vi "SetZForInte_modify_Bmode_temperature_PRF&Volt.vi"(6 "meas_setting":T3={"measSetId"=6949, "measSetComments"="Orchid", "probeId"=141.0, "beamstyleIndex"=0, "txFrequencyHz"=3636400.0, "focusRangeCm"=8.0, "maxTxVoltageVolt"=100.0, "ceilTxVoltageVolt"=80.0, "profTxVoltageVolt"=62.0, "totalVoltagePt"=20, "numMeasVoltage"=12, "numTxElements"=118, "txpgWaveformStyle"=2, "numTxCycles"=4.0, "elevAperIndex"=0, "zStartDistCm"=1.5, "zMeasNum"=80, "IsTxAperModulationEn"=0, "DTxFreqIndex"=0, "VTxIndex"=0, "IsCPAEn"=0, "SysPulserSelA"=0, "TxPulseRleA"=""} {"zStartDistCm" format="%.2f"; "numTxCycles" format="%.1f"; "profTxVoltageVolt" format="%#_1g"; "ceilTxVoltageVolt" format="%.2f"; "maxTxVoltageVolt" format="%.2f"; "focusRangeCm" format="%.1f"; "txFrequencyHz" format="%.2f"}, 7 "timeout (ms)":dbl=40000.0 format="%.2f", 8 "error in (no error)":errorcluster, 9 "CW":bool, 10 "meas_temparature_Input":T2 {"scanRange" format="%.2f"; "numTxCycles" format="%#.2f"; "temperatureC" format="%.2f"; "pulseVoltage" format="%.2f"; "roomTempC" format="%.2f"}, 11 "TCP from Orchid in":refnum<k5>) -> (0 "error out":errorcluster, 1 "veri_P/F":bool, 2 "meas_temparature_Output":T1 {"scanRange" format="%.2f"; "temperatureC" format="%.2f"; "pulseVoltage" format="%.2f"; "roomTempC" format="%.2f"}, 3 "Actual PRF":dbl)   [LabVIEW 2016]
doc: "This VI sets the Z system transmit parameters for an intensity measurement, reads them back, and checks for errors. It first gets the initial center element delay (TxpgDelayAperA) and the system frequencies using tcpSysTxFreqFromZ.vi. It then sets the elevation aperture (using SetZElevAper.vi), channel modulation, wavestyle, frequency, focus, number of transmit elements, number of cycles, voltage, and voltage channel, in that order. It reads back the settings (using tcpReadIntenSettingsZ.vi) and checks for errors. The final trigger delay and change in delay, in microseconds, are calculated from the initial and final values of TxpgDelayAperA using:\ndelay(us) = (TxpgDelayAperA + 178.0) / 160"
uses:
  type def/measSetting.ctl
  GrobaLimitVoltage.vi
  TemperatureMeasure/Thermal_type.vi
panel:
  out "Receive array":string[](array[string])=["\r\n220 OK\r\nContainers within Hardware Control Layer\r\n\tHardwareModel\r\n\tHardwareControl\r\n\tHardwareAlgorithm\r\n\tSeq\r\n\tBeamforming\r\n\tDigitalReceiver\r\n\tEchoProcessor\r\n\tFlowProcessor\r\n\tHardwareScanConverter\r\n\tSip\r\n\tVideoInterface\r\n\tRtc\r\n\tCine\r\nScalar Parameters of Hardware Control Layer\r\nArray Parameters of Hardware Control Layer\r\ndebug\tDebug Functions\r\nquit\tExit DIOS\r\nback\tPrevious menu\r\nmain\tTop menu\r\nhelp\tAvailable commands\r\n\r\n", "\r\n220 OK\r\nContainers within Beamforming\r\n\tCommon\r\n\tBImage\r\n\tCbImage\r\n\tDImage\r\nScalar Parameters of Beamforming\r\nArray Parameters of Beamforming\r\ndebug\tDebug Functions\r\nquit\tExit DIOS\r\nback\tPrevious menu\r\nmain\tTop menu\r\nhelp\tAvailable commands\r\n\r\n", "\r\n220 OK\r\nContainers within Common\r\nScalar Parameters of Common\r\n\tBfPropagationVelCmPerSec\t154000\r\n\tDisUnit\t0.00385\r\n\tHwRcInterruptMask\t63\r\n\tHwRcTVP\t3\r\n\tHwRxAac0\t175\r\n\tHwRxAac1\t0\r\n\tHwRxbfBlankingWord\t0\r\n\tHwRxbfCmd1Word\t4232\r\n\tHwRxbfCmd2Word\t2\r\n\tHwRxbf0Cmd2Word\t3\r\n\tHwRxbfStartDelayWord\t10\r\n\tHwTiAttenuatorSelect\t0\r\n\tHwTiBitEn\t25088\r\n\tHwTiDacCtrl0\t255\r\n\tHwTiDacCtrl1\t2303\r\n\tHwTiDacCtrl2\t3327\r\n\tHwTiDacCtrl3\t511\r\n\tHwTiDacCtrl4\t2559\r\n\tHwTiDacCtrl5\t3583\r\n\tHwTiDacCtrl6\t767\r\n\tHwTiDacCtrl7\t2815\r\n\tHwTiDacCtrl8\t3839\r\n\tHwTiDacCtrl9\t2047\r\n\tHwTiDacCtrl10\t4095\r\n\tHwTiDigitalDriveCtrl\t0\r\n\tHwTiDigitalInterruptPolarity\t0\r\n\tHwTiDigitalReadCtrl\t0\r\n\tHwTiEchoBoosterCtrl\t0\r\n\tHwTiGlobalCtrl\t1\r\n\tHwTiHighVoltEn\t0\r\n\tHwTiInterruptClear\t65535\r\n\tHwTiInterruptMask\t32767\r\n\tHwTiMiscBitCtrl\t12\r\n\tHwTiProbeSelect\t2\r\n\tHwTiTXCLTransfer\t0\r\n\tHwTiVoltMultiplexer\t0\r\n\tHwTrGlobalCtrlAll\t1\r\n\tHwTrGlobalCtrl0All\t0\r\n\tHwTrDiagnosticCtrlAll\t0\r\n\tHwTrInterruptMaskAll\t1\r\n\tHwTrInterruptClearAll\t1\r\n\tHwTrRealTimeCtrlAll\t40\r\n\tHwTrTgcAacSignalCtrlAll\t0\r\n\tRxDelayRefx\t1\r\n\tRxDelayRefy\t-1\r\n\tTrPartNumber\t5928150\r\n\tBfPropagationVelFactor\t1\r\n\tDigitizingRateHz\t4e+007\r\n\tHwRxBfVectorLengthWord\t0\r\n\tIsRxVectorLengthEn\t1\r\n\tNumChannels\t192\r\n\tProbeBandwidthHz\t3.6e+006\r\n\tProbeId\t171\r\n\tProbeNumElem\t192\r\n\tProbeNumRows\t1\r\n\tProbePitchCm\t0.02\r\n\tProbeRadiusElectricalCm\t0\r\n\tProbeType\t0\r\n\tPropagationVelCmPerSec\t154000\r\n\tRxApod2dEn\t0\r\n\tRxbfAdcDelayClocks\t10\r\n\tRxbfGainShift\t0\r\n\tRxDelayYOffsetSysClk4\t0\r\n\tTxPulserMaxVolt\t50\r\nArray Parameters of Common\r\n\tHwRxbf0AdGainA\tsize=64\r\n\tHwRxbf1AdGainA\tsize=64\r\n\tHwRxbf2AdGainA\tsize=64\r\n\tHwRxbf3AdGainA\tsize=64\r\n\tHwRxbf4AdGainA\tsize=64\r\n\tHwRxbf5AdGainA\tsize=64\r\n\tHwRxbf6AdGainA\tsize=64\r\n\tHwRxbf7AdGainA\tsize=64\r\n\tHwRxbf8AdGainA\tsize=64\r\n\tHwRxbf9AdGainA\tsize=64\r\n\tHwRxbf10AdGainA\tsize=64\r\n\tHwRxbf11AdGainA\tsize=64\r\n\tHwRxAdOffsetCalA\tsize=192\r\n\tHwRxApodFilterRamA\tsize=512\r\n\tHwRxbf0DelayCalA\tsize=64\r\n\tHwRxbf1DelayCalA\tsize=64\r\n\tHwRxbf2DelayCalA\tsize=64\r\n\tHwRxbf3DelayCalA\tsize=64\r\n\tHwRxbf4DelayCalA\tsize=64\r\n\tHwRxbf5DelayCalA\tsize=64\r\n\tHwRxbf6DelayCalA\tsize=64\r\n\tHwRxbf7DelayCalA\tsize=64\r\n\tHwRxbf8DelayCalA\tsize=64\r\n\tHwRxbf9DelayCalA\tsize=64\r\n\tHwRxbf10DelayCalA\tsize=64\r\n\tHwRxbf11DelayCalA\tsize=64\r\n\tHwRxbf0DxA\tsize=64\r\n\tHwRxbf1DxA\tsize=64\r\n\tHwRxbf2DxA\tsize=64\r\n\tHwRxbf3DxA\tsize=64\r\n\tHwRxbf4DxA\tsize=64\r\n\tHwRxbf5DxA\tsize=64\r\n\tHwRxbf6DxA\tsize=64\r\n\tHwRxbf7DxA\tsize=64\r\n\tHwRxbf8DxA\tsize=64\r\n\tHwRxbf9DxA\tsize=64\r\n\tHwRxbf10DxA\tsize=64\r\n\tHwRxbf11DxA\tsize=64\r\n\tHwRxbf0DyA\tsize=64\r\n\tHwRxbf1DyA\tsize=64\r\n\tHwRxbf2DyA\tsize=64\r\n\tHwRxbf3DyA\tsize=64\r\n\tHwRxbf4DyA\tsize=64\r\n\tHwRxbf5DyA\tsize=64\r\n\tHwRxbf6DyA\tsize=64\r\n\tHwRxbf7DyA\tsize=64\r\n\tHwRxbf8DyA\tsize=64\r\n\tHwRxbf9DyA\tsize=64\r\n\tHwRxbf10DyA\tsize=64\r\n\tHwRxbf11DyA\tsize=64\r\n\tHwRxbf0DzA\tsize=128\r\n\tHwRxbf1DzA\tsize=128\r\n\tHwRxbf2DzA\tsize=128\r\n\tHwRxbf3DzA\tsize=128\r\n\tHwRxbf4DzA\tsize=128\r\n\tHwRxbf5DzA\tsize=128\r\n\tHwRxbf6DzA\tsize=128\r\n\tHwRxbf7DzA\tsize=128\r\n\tHwRxbf8DzA\tsize=128\r\n\tHwRxbf9DzA\tsize=128\r\n\tHwRxbf10DzA\tsize=128\r\n\tHwRxbf11DzA\tsize=128\r\n\tHwRxbf0PosInApodWinA\tsize=64\r\n\tHwRxbf1PosInApodWinA\tsize=64\r\n\tHwRxbf2PosInApodWinA\tsize=64\r\n\tHwRxbf3PosInApodWinA\tsize=64\r\n\tHwRxbf4PosInApodWinA\tsize=64\r\n\tHwRxbf5PosInApodWinA\tsize=64\r\n\tHwRxbf6PosInApodWinA\tsize=64\r\n\tHwRxbf7PosInApodWinA\tsize=64\r\n\tHwRxbf8PosInApodWinA\tsize=64\r\n\tHwRxbf9PosInApodWinA\tsize=64\r\n\tHwRxbf10PosInApodWinA\tsize=64\r\n\tHwRxbf11PosInApodWinA\tsize=64\r\n\tHwRxMuxSelectLutA\tsize=512\r\n\tHwRxRamOffsetA\tsize=12\r\n\tHwTxDacA\tsize=2\r\n\tHwTxpgDelayAperA\tsize=393216\r\n\tNumBitsPerCycleA\tsize=49\r\n\tNumCyclesPerPassA\tsize=49\r\n\tNumWordsPerPassA\tsize=49\r\n\tRxAdGainA\tsize=256\r\n\tRxDelayCalA\tsize=768\r\n\tRxDxA\tsize=256\r\n\tRxDyA\tsize=256\r\n\tRxDzA\tsize=256\r\n\tRxMuxSelectLutPtrA\tsize=512\r\n\tRxPosInApodWinA\tsize=768\r\n\tTxDelayCalA\tsize=192\r\n\tTxpgWaveformHoutA\tsize=15680\r\n\tTxpgWaveformLoutA\tsize=15680\r\n\tYIndexTableA\tsize=256\r\n\tZIndexTableA\tsize=256\r\n\tInsertedProbeIdA\tsize=6\r\n\tPulseVoltageA\tsize=2\r\n\tRxApodFactorA\tsize=4\r\n\tRxApodSelA\tsize=4\r\n\tSysTxFreqHzA\tsize=49\r\ndebug\tDebug Functions\r\nquit\tExit DIOS\r\nback\tPrevious menu\r\nmain\tTop menu\r\nhelp\tAvailable commands\r\n\r\n", "220 OK\r\n", "250 20\r\n"]
  out "error out 2":errorcluster
  out "Pass_count":i16
  out "All_param_veri":bool[](array[boolean])
  in  "volt channel":i8
  # "Program constants"
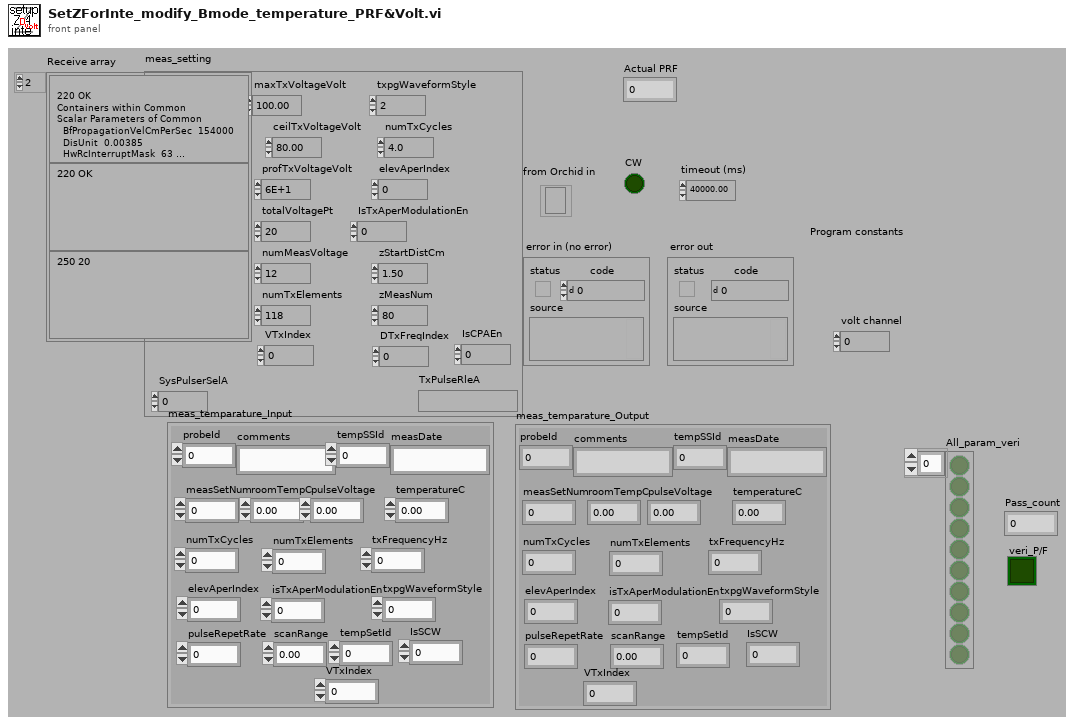
[diagram p1: front panel]
types:
  T1 = cluster{"probeId":sgl, "comments":string, "tempSSId":i16, "measDate":string, "measSetNum":i16, "roomTempC":sgl, "pulseVoltage":dbl, "temperatureC":ext, "numTxCycles":dbl, "numTxElements":i16, "txFrequencyHz":i32, "elevAperIndex":i16, "isTxAperModulationEn":i16, "txpgWaveformStyle":i16, "pulseRepetRate":i32, "scanRange":dbl, "tempSetId":i16, "IsSCW":i16, "VTxIndex":i16}
  T2 = cluster{"probeId":sgl, "comments":string, "tempSSId":i16, "measDate":string, "measSetNum":i16, "roomTempC":sgl, "pulseVoltage":dbl, "temperatureC":ext, "numTxCycles":dbl, "numTxElements":i16, "txFrequencyHz":i32, "elevAperIndex":i16, "isTxAperModulationEn":i16, "txpgWaveformStyle":i16, "pulseRepetRate":dbl, "scanRange":dbl, "tempSetId":i16, "IsSCW":i16, "VTxIndex":i16}
  T3 = typedef "measSetting.ctl" = cluster{"measSetId":i32, "measSetComments":string, "probeId":sgl, "beamstyleIndex":i16, "txFrequencyHz":sgl, "focusRangeCm":sgl, "maxTxVoltageVolt":sgl, "ceilTxVoltageVolt":sgl, "profTxVoltageVolt":dbl, "totalVoltagePt":i8, "numMeasVoltage":i8, "numTxElements":i16, "txpgWaveformStyle":i8, "numTxCycles":sgl, "elevAperIndex":i8, "zStartDistCm":sgl, "zMeasNum":i8, "IsTxAperModulationEn":i8, "DTxFreqIndex":i16, "VTxIndex":i8, "IsCPAEn":i16, "SysPulserSelA":i16, "TxPulseRleA":string}
  T4 = cluster{"pulseVoltage":dbl, "numTxCycles":dbl, "numTxElements":i16, "txFrequencyIndex":i32, "isTxAperModulationEn":i16, "txpgWaveformStyle":i16, "pulseRepetRate":dbl, "FocalRangeCm":dbl, "RoiLateralSpan":dbl, "RoiLateralMin":dbl}
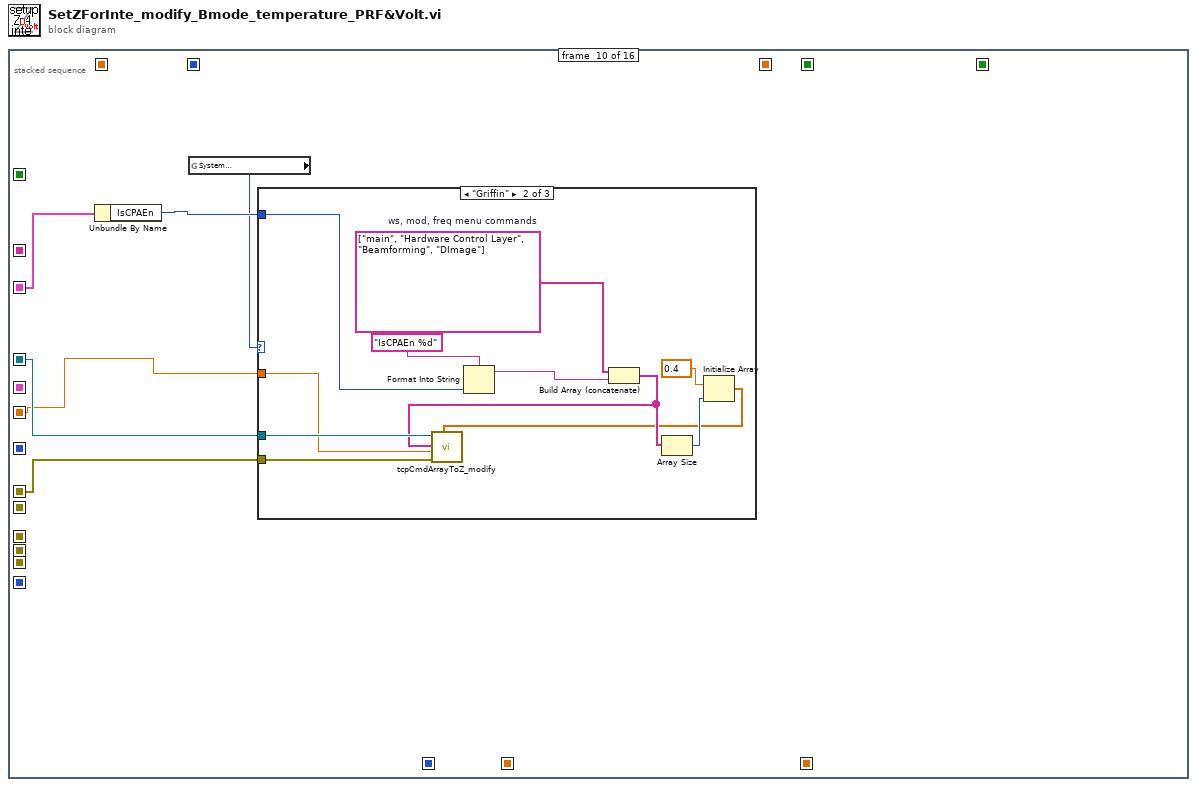
[diagram p0: block diagram]
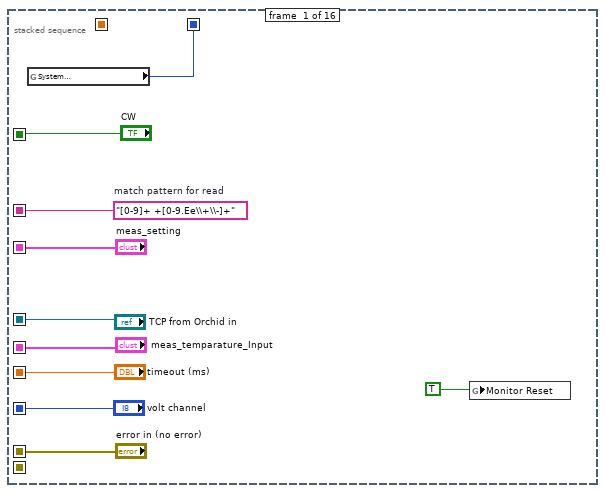
[diagram p2: hidden frame]
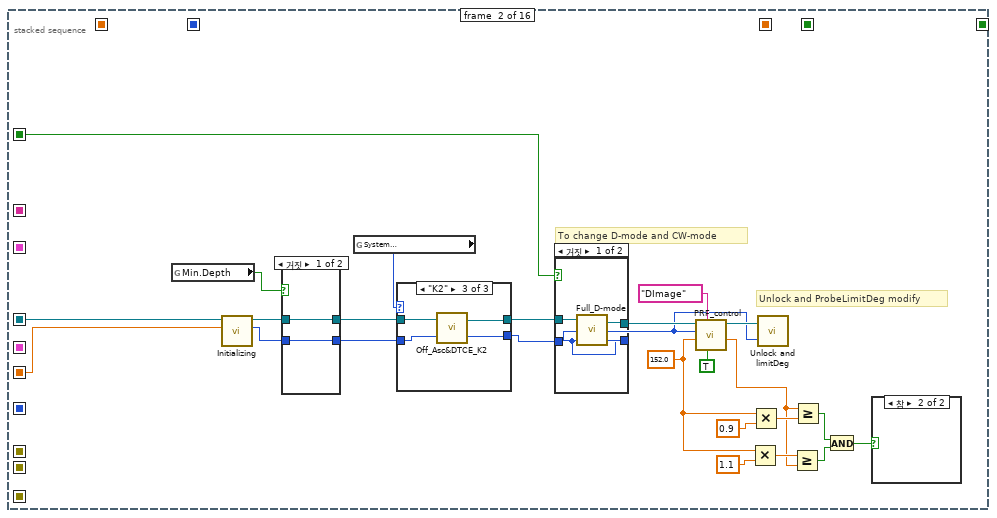
[diagram p3: hidden frame]
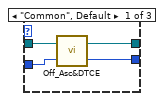
[diagram p4: hidden frame]
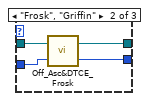
[diagram p5: hidden frame]
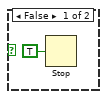
[diagram p6: hidden frame]
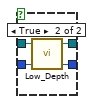
[diagram p7: hidden frame]
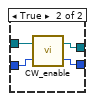
[diagram p8: hidden frame]
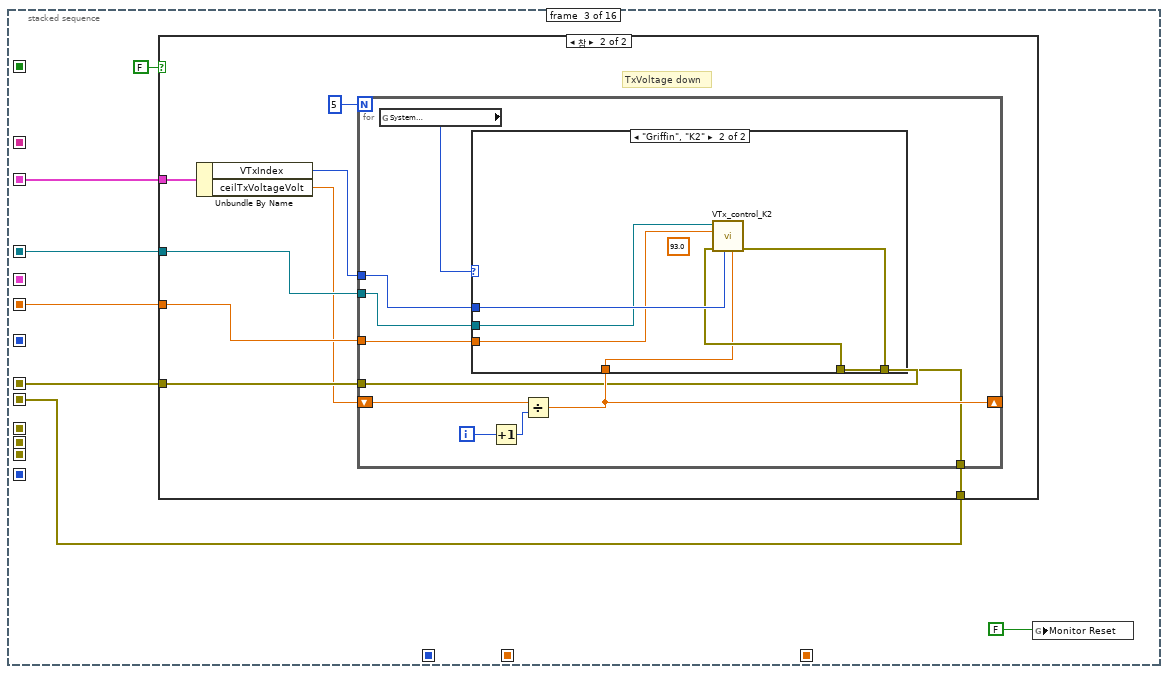
[diagram p9: hidden frame]
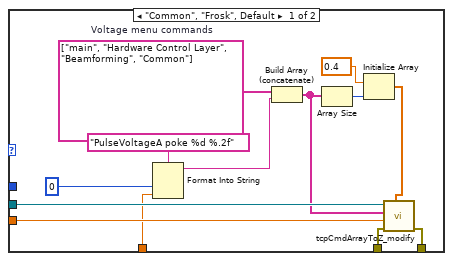
[diagram p11: hidden frame]
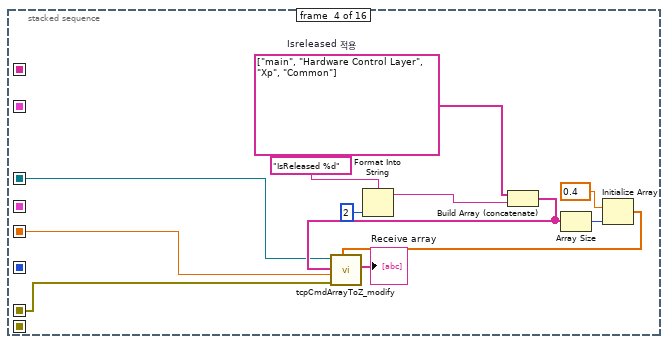
[diagram p12: hidden frame]
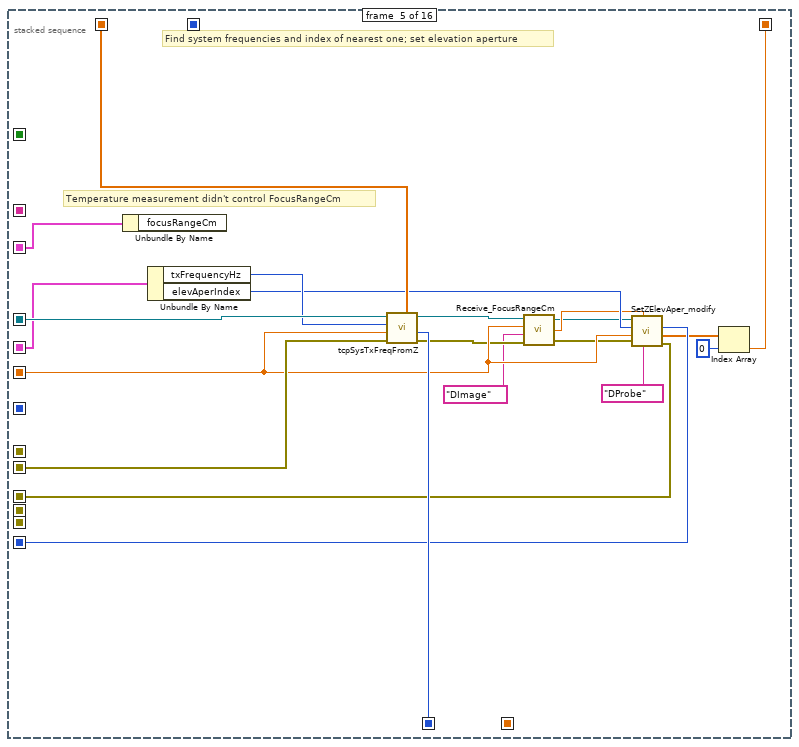
[diagram p13: hidden frame]
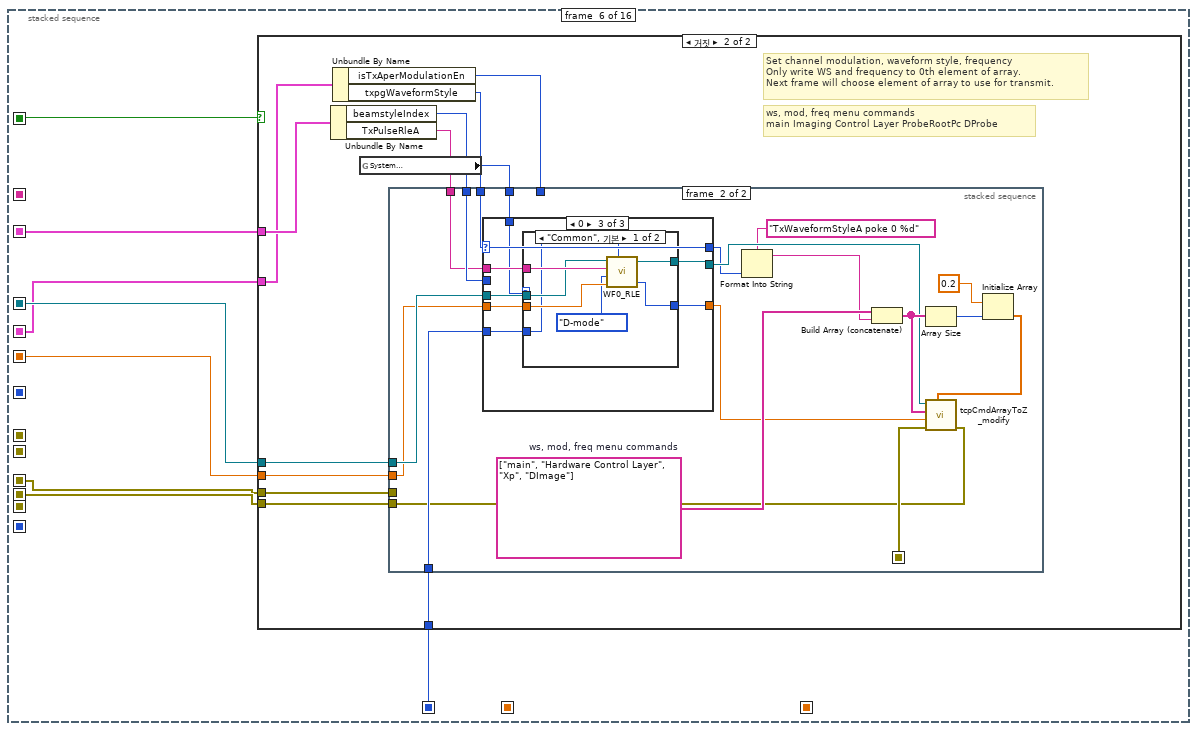
[diagram p14: hidden frame]
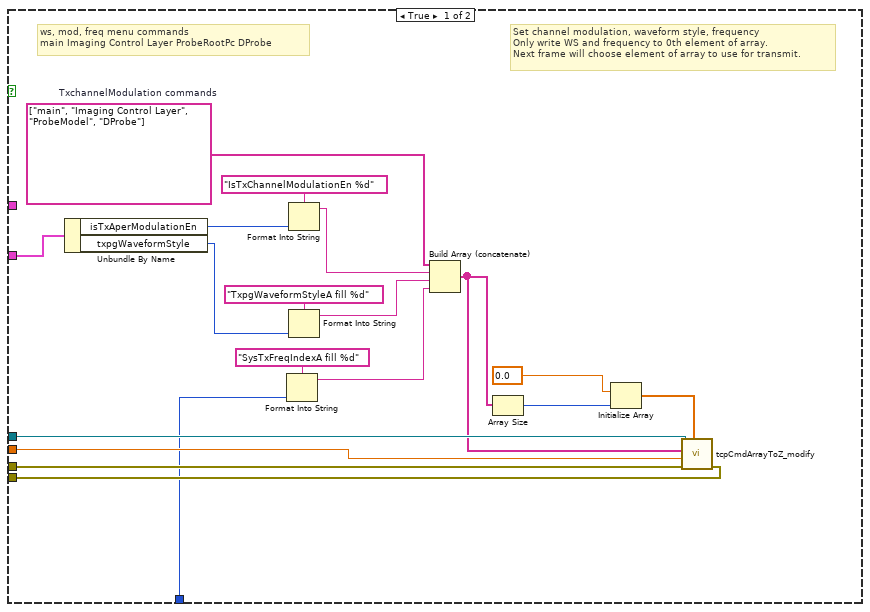
[diagram p15: hidden frame]
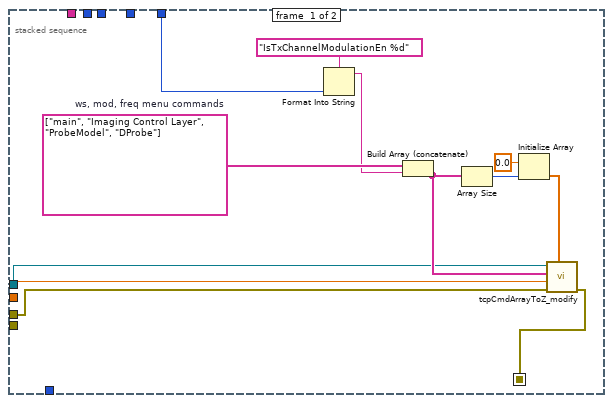
[diagram p16: hidden frame]
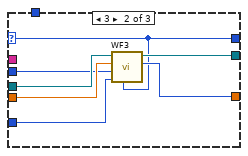
[diagram p18: hidden frame]
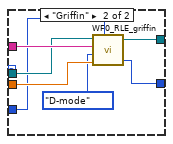
[diagram p19: hidden frame]
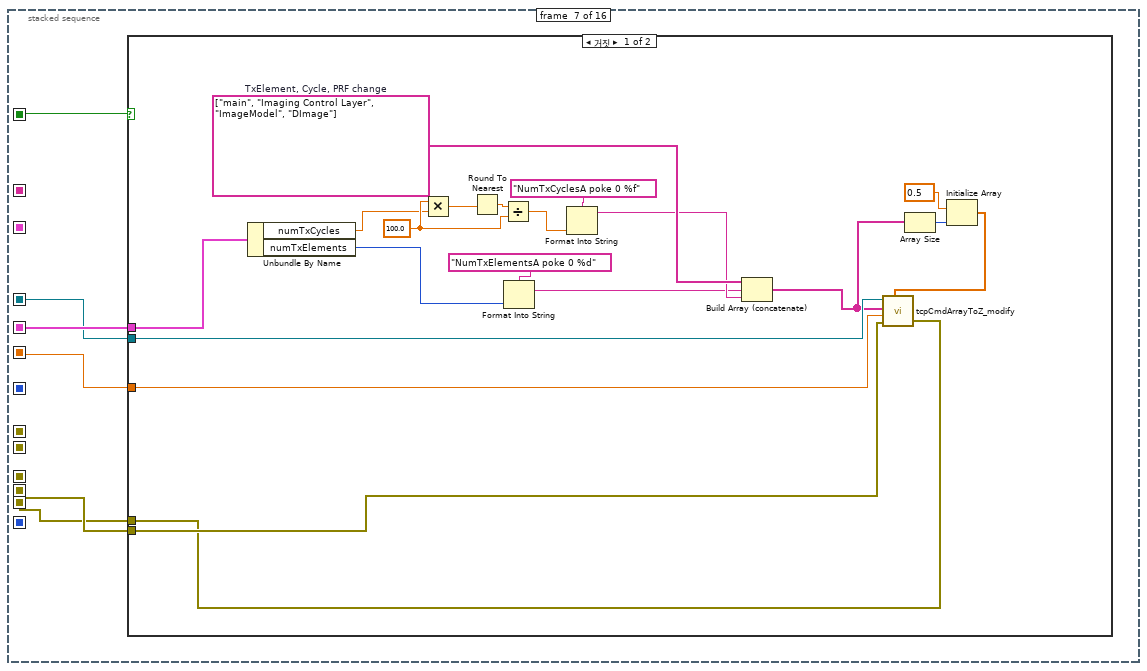
[diagram p20: hidden frame]
diagram:
  n1 = stacked-sequence {
    seq-local: ["meas_temparature_Input" _ _ _ _ _ _ _ _ _ _ _ _ _ _ _] -> [_ _ _ _ w138 w142 w247 w293 _ _ _ w394 w465 _ _ _]
    seq-local: ["TCP from Orchid in" _ _ _ _ _ _ _ _ _ _ _ _ _ _ _] -> [_ w35 w68 w109 w139 w147 w245 w281 w296 w311 w339 w396 w458 w509 w518 w525]
    seq-local: ["timeout (ms)" _ _ _ _ _ _ _ _ _ _ _ _ _ _ _] -> [_ w34 w67 w107 w124 w146 w244 w279 w295 w310 w337 w395 w457 w508 w517 w524]
    seq-local: [_ _ _ _ w133 _ _ _ _ _ _ _ _ _ _ _] -> [_ _ _ _ _ w144 _ _ _ _ _ _ _ _ _ _]
    seq-local: [_ _ _ _ w137 _ _ _ _ _ _ _ _ _ _ _] -> [_ _ _ _ _ _ _ _ _ _ _ _ _ _ _ _]
    seq-local: ["volt channel" _ _ _ _ _ _ _ _ _ _ _ _ _ _ _] -> [_ _ _ _ _ _ _ _ _ _ _ _ _ _ _ _]
    seq-local: ["error in (no error)" _ _ _ _ _ _ _ _ _ _ _ _ _ _ _] -> [_ _ w64 w108 _ _ _ _ _ w309 w338 w414 _ _ _ _]
    seq-local: [w7 _ _ _ _ _ _ _ _ _ _ _ _ _ _ _] -> [_ _ _ _ _ _ _ _ _ _ _ _ _ _ _ _]
    seq-local: [_ _ w63 _ _ _ _ _ _ _ _ _ _ _ _ _] -> [_ _ _ _ w134 _ _ _ _ _ _ _ _ _ _ _]
    seq-local: [_ _ _ _ _ w145 _ _ _ _ _ _ _ _ _ _] -> [_ _ _ _ _ _ w246 _ _ _ _ _ _ _ _ _]
    seq-local: [_ _ _ _ _ _ w243 _ _ _ _ _ _ _ _ _] -> [_ _ _ _ _ _ _ _ _ _ _ _ w456 w504 _ _]
    seq-local: ["meas_setting" _ _ _ _ _ _ _ _ _ _ _ _ _ _ _] -> [_ _ w66 _ w126 w140 _ _ _ w308 _ w393 w460 _ _ _]
    seq-local: ["CW" _ _ _ _ _ _ _ _ _ _ _ _ _ _ _] -> [_ w31 _ _ _ w143 w242 _ _ _ _ w397 w451 _ _ _]
    seq-local: [_ _ _ _ w135 _ _ _ _ _ _ _ _ _ _ _] -> [_ _ _ _ _ w141 _ _ w297 _ _ w412 _ _ _ _]
    seq-local: [_ _ _ _ _ _ _ _ _ _ _ w386 _ _ _ _] -> [_ _ _ _ _ _ _ _ _ _ _ _ _ w507 _ _]
    seq-local: [_ _ _ _ _ _ _ w280 _ _ _ _ _ _ _ _] -> [_ _ _ _ _ _ _ _ _ _ _ w413 _ _ _ _]
    seq-local: [_ _ _ _ _ _ _ _ _ _ _ _ w453 _ _ _] -> [_ _ _ _ _ _ _ _ _ _ _ _ _ w506 _ _]
    seq-local: [_ _ _ _ w130 _ _ _ _ _ _ _ _ _ _ _] -> [_ _ _ _ _ _ _ _ _ _ _ w385 _ _ _ _]
    seq-local: [_ _ _ _ w127 _ _ _ _ _ _ _ _ _ _ _] -> [_ _ _ _ _ _ _ _ _ _ _ w384 _ _ _ _]
    seq-local: [w1 _ _ _ _ _ _ _ _ _ _ _ _ _ _ _] -> [_ _ _ _ _ _ _ _ w294 _ _ w390 w452 _ _ _]
    seq-local: [_ _ _ _ _ _ _ _ _ _ w335 _ _ _ _ _] -> [_ _ _ _ _ _ _ _ _ _ _ w367 _ _ _ _]
    frame #0 {
      w7 = "[0-9]+ +[0-9.Ee\\+\\-]+"  # match pattern for read
      n2 = global read "Thermal_type.vi" "System \nSelection"() -> (w1:enum32{"Common", "Frosk", "Griffin", "K2"})
      n3 = global write "GrobaLimitVoltage.vi" "Monitor Reset"(TRUE) -> ()
    }
    frame #1 {
      w20 = 152.0 ("Input PRF")
      # "Unlock and ProbeLimitDeg modify"
      # "To change D-mode and CW-mode"
      n4 = global read "Thermal_type.vi" "Min.Depth"() -> (w30:bool)
      n5 = call "Initializing.vi"("Timeout (ms)"=w34, "connection ID in"=w35) -> ("Timeout (ms) 2"=w32:i32, "connection ID in 2"=w33:refnum<k5>)  [unwired: 8 in]
      n6 = case shown="거짓" w30 {
        tunnel: w33 -> [w50 w54]
        tunnel: w32 -> [w49 w53]
        tunnel: [w50 w52] -> w14
        tunnel: [w49 w51] -> w13
        frame False {
        }
        frame True {
          n7 = call "Low_Depth.vi"("Timeout (ms)"=w53, "connection ID in"=w54) -> ("Timeout (ms) 2"=w51:i32, "connection ID out"=w52:refnum<k5>)  [unwired: 2 in]
        }
      }
      n8 = global read "Thermal_type.vi" "System \nSelection"() -> (w15:enum32{"Common", "Frosk", "Griffin", "K2"})
      n9 = case shown="\"K2\"" w15 {
        tunnel: [w39 w43 w45] -> w12
        tunnel: [w38 w42 w44] -> w11
        tunnel: w14 -> [w37 w41 w47]
        tunnel: w13 -> [w36 w40 w46]
        frame "Common", Default {
          n10 = call "Off_Asc&DTCE.vi"("Timeout (ms)"=w36, "connection ID in"=w37) -> ("Timeout (ms) 2"=w38:i32, "connection ID out"=w39:refnum<k5>)
        }
        frame "Frosk", "Griffin" {
          n11 = call "Off_Asc&DTCE_Frosk.vi"("Timeout (ms)"=w40, "connection ID in"=w41) -> ("Timeout (ms) 2"=w42:i32, "connection ID out"=w43:refnum<k5>)
        }
        frame "K2" {
          n12 = call "Off_Asc&DTCE_K2.vi"("Timeout (ms)"=w46, "connection ID in"=w47) -> ("Timeout (ms) 2"=w44:i32, "connection ID out"=w45:refnum<k5>)
        }
      }
      n13 = case shown="거짓" w31 {
        tunnel: w12 -> [w57 w61]
        tunnel: w11 -> [w55 w60]
        tunnel: [w56 w59] -> w19
        tunnel: [w55 w58] -> w17
        frame False {
          n14 = call "Full_D-mode.vi"("Timeout (ms) 입력"=w55, "TCP 네트워크 연결 입력"=w57) -> ("TCP 네트워크 연결 출력"=w56:refnum<k5>)  [unwired: 1 in]
        }
        frame True {
          n15 = call "CW_enable.vi"("Timeout (ms)"=w60, "connection ID in"=w61) -> ("Timeout (ms) 2"=w58:i32, "connection ID out"=w59:refnum<k5>)
        }
      }
      n16 = call "PRF_control.vi"("PRF_Event Down"=TRUE, "mode selection"="DImage", "Input PRF"=w20, "timeout (ms)"=w17, "TCP from Orchid in"=w19) -> ("PRF"=w21:dbl, "connection ID out"=w18:refnum<k5>)  [unwired: 2 in, 1 out]
      n17 = Multiply(x=w20, y=1.1) -> (x*y=w26:dbl)
      n18 = Multiply(x=w20, y=0.9) -> (x*y=w22:dbl)
      n19 = call "Unlock and limitDeg.vi"("Timeout (ms)"=w17, "connection ID in"=w18) -> ()  [unwired: 2 out]
      n20 = Greater Or Equal?(x=w26, y=w21) -> (x >= y?=w25:bool)
      n21 = Greater Or Equal?(x=w21, y=w22) -> (x >= y?=w24:bool)
      n22 = And(x=w24, y=w25) -> (x .and. y?=w23:bool)
      n23 = case shown="참" w23 {
        frame False {
          n24 = Stop(stop? (T)=TRUE ("정지? (참)")) -> ()
        }
        frame True {
        }
      }
    }
    frame #2 {
      n25 = case shown="참" FALSE {
        tunnel: w68 -> [_ w77]
        tunnel: w67 -> [_ w76]
        tunnel: w66 -> [_ w75]
        tunnel: w64 -> [w69 w72]
        tunnel: [w69 w71] -> w63
        frame False {
        }
        frame True {
          # "TxVoltage down"
          n26 = Unbundle By Name(w75) -> ("VTxIndex"=w73:i8, "ceilTxVoltageVolt"=w70:sgl)
          n27 = for {
            N: 5 -> [_]
            tunnel: w77 -> [w87]
            tunnel: w76 -> [w86]
            shift-right: [w80] -> _
            shift-left: w70 -> [w82]
            tunnel: w73 -> [w85]
            tunnel: w72 -> [w79]
            tunnel: [w78] -> w71
            i -> [w81]
            n28 = global read "Thermal_type.vi" "System \nSelection"() -> (w84:enum32{"Common", "Frosk", "Griffin", "K2"})
            n29 = Increment(x=w81) -> (x+1=w83:i32)
            n30 = Divide(x=w82, y=w83) -> (x/y=w80:sgl)
            n31 = case shown="\"Griffin\", \"K2\"" w84 {
              tunnel: w87 -> [w100 w105]
              tunnel: w86 -> [w99 w104]
              tunnel: w85 -> [_ w106]
              tunnel: w80 -> [w90 w101]
              tunnel: w79 -> [w89 w103]
              tunnel: [w88 w102] -> w78
              frame "Common", "Frosk", Default {
                w97 = string[] ["main", "Hardware Control Layer", "Beamforming", "Common"]  # Voltage menu commands
                n32 = Format Into String(format string="PulseVoltageA poke %d %.2f" ("Format String"), i8 0 ("입력 1"), w90) -> (resulting string=w96:string)  [unwired: 2 in, 1 out]
                n33 = Build Array (concatenate)(w97, w96) -> (w92:string[])
                n34 = Array Size(array=w92) -> (size(s)=w95:i32)
                n35 = Initialize Array(0.4 ("element"), w95) -> (w93:dbl[])
                n36 = call "tcpCmdArrayToZ_modify.vi"("Delay (sec)"=w93, "error in (no error)"=w89, "Timeout (ms)"=w99, "Command array"=w92, "connection ID in"=w100) -> ("error out"=w88:errorcluster)  [unwired: 2 in, 4 out]
              }
              frame "Griffin", "K2" {
                (unwired) 93.0 ("VTx1_voltage")
                n37 = call "VTx_control_K2.vi"("VTx_Voltage"=w101, "VTxIndex_In"=w106, "error in (no error)"=w103, "Timeout (ms)"=w104, "connection ID in"=w105) -> ("error out"=w102:errorcluster)  [unwired: 5 in, 1 out]
              }
            }
          }
        }
      }
      n38 = global write "GrobaLimitVoltage.vi" "Monitor Reset"(FALSE) -> ()
    }
    frame #3 {
      w112 = string[] ["main", "Hardware Control Layer", "Xp", "Common"]  # Isreleased 적용
      n39 = Format Into String(format string="IsReleased %d" ("Format String"), i16 2 ("입력 1")) -> (resulting string=w117:string)  [unwired: 2 in, 1 out]
      n40 = Build Array (concatenate)(w112, w117) -> (w114:string[])
      n41 = Array Size(array=w114) -> (size(s)=w116:i32)
      n42 = Initialize Array(0.4 ("element"), w116) -> (w113:dbl[])
      n43 = call "tcpCmdArrayToZ_modify.vi"("Delay (sec)"=w113, "error in (no error)"=w108, "Timeout (ms)"=w107, "Command array"=w114, "connection ID in"=w109) -> ("Receive array"=→"Receive array":string[])  [unwired: 2 in, 4 out]
    }
    frame #4 {
      # "Temperature measurement didn't control FocusRangeCm"
      # "Find system frequencies and index of nearest one; set elevation aperture"
      n44 = Unbundle By Name(w126) -> ()  [unwired: 1 out]
      n45 = Unbundle By Name(w138) -> ("txFrequencyHz"=w136:i32, "elevAperIndex"=w132:i16)
      n46 = call "tcpSysTxFreqFromZ.vi"("error in (no error)"=w134, "timeout (ms)"=w124, "txFrequencyHz in"=w136, "connection ID in"=w139) -> ("error out"=w123:errorcluster, "TxFreqIndex"=w135:i8, "connection ID out"=w121:refnum<k5>, "SysTxFreqHzA"=w137:sgl[])  [unwired: 3 in, 1 out]
      n47 = call "Receive_FocusRangeCm.vi"("error in (no error)"=w123, "Image mode"="DImage", "Timeout (ms)"=w124, "connection ID in"=w121) -> ("error out"=w122:errorcluster, "FocusRangeCm"=w125:dbl, "connection ID out"=w120:refnum<k5>)
      n48 = call "SetZElevAper_modify.vi"("Mode"="DProbe", "focusRangeCm"=w125, "error in (no error)"=w122, "timeout (ms)"=w124, "elevAperIndex"=w132, "connection ID in"=w120) -> ("error out"=w133:errorcluster, "SwitchDepth"=w129:sgl[], "probeNumElevAper"=w130:i32)  [unwired: 2 in, 1 out]
      n49 = Index Array(array=w129, index=0 ("인덱스")) -> (element=w127:sgl)
    }
    frame #5 {
      n50 = case shown="거짓" w143 {
        tunnel: w147 -> [w166 w176]
        tunnel: w146 -> [w165 w175]
        tunnel: [w163 w169] -> w145
        tunnel: w144 -> [w162 w178]
        tunnel: w142 -> [w160 w173]
        tunnel: w141 -> [w149 w177]
        tunnel: w140 -> [_ w174]
        frame True {
          w155 = string[] ["main", "Imaging Control Layer", "ProbeModel", "DProbe"]  # TxchannelModulation commands
          # "ws, mod, freq menu commands\nmain Imaging Control Layer ProbeRootPc DProbe"
          # "Set channel modulation, waveform style, frequency\nOnly write WS and frequency to 0th element of array.\nNext frame will choose element of array to use for transmit."
          n51 = Unbundle By Name(w160) -> ("isTxAperModulationEn"=w161:i16, "txpgWaveformStyle"=w153:i16)
          n52 = Format Into String(format string="SysTxFreqIndexA fill %d" ("Format String"), w149) -> (resulting string=w148:string)  [unwired: 2 in, 1 out]
          n53 = Format Into String(format string="IsTxChannelModulationEn %d" ("Format String"), w161) -> (resulting string=w154:string)  [unwired: 2 in, 1 out]
          n54 = Format Into String(format string="TxpgWaveformStyleA fill %d" ("Format String"), w153) -> (resulting string=w152:string)  [unwired: 2 in, 1 out]
          n55 = Build Array (concatenate)(w155, w154, w152, w148) -> (w159:string[])
          n56 = Array Size(array=w159) -> (size(s)=w158:i32)
          n57 = Initialize Array(0.0 ("element"), w158) -> (w156:dbl[])
          n58 = call "tcpCmdArrayToZ_modify.vi"("Delay (sec)"=w156, "error in (no error)"=w162, "Timeout (ms)"=w165, "Command array"=w159, "connection ID in"=w166) -> ("error out"=w163:errorcluster)  [unwired: 2 in, 4 out]
        }
        frame False {
          # "ws, mod, freq menu commands\nmain Imaging Control Layer ProbeRootPc DProbe"
          # "Set channel modulation, waveform style, frequency\nOnly write WS and frequency to 0th element of array.\nNext frame will choose element of array to use for transmit."
          n59 = Unbundle By Name(w174) -> ("beamstyleIndex"=w170:i16, "TxPulseRleA"=w168:string)
          n60 = Unbundle By Name(w173) -> ("isTxAperModulationEn"=w172:i16, "txpgWaveformStyle"=w171:i16)
          n61 = global read "Thermal_type.vi" "System \nSelection"() -> (w167:enum32{"Common", "Frosk", "Griffin", "K2"})
          n62 = stacked-sequence {
            seq-local: [w179 _] -> [_ w195]
            tunnel: w178 -> [w180 _]
            tunnel: w177 -> [_ w199]
            tunnel: w176 -> [w183 w204]
            tunnel: w175 -> [w182 w201]
            tunnel: w172 -> [w181 _]
            tunnel: w171 -> [_ w193]
            tunnel: w170 -> [_ w200]
            tunnel: [_ w194] -> w169
            tunnel: w168 -> [_ w192]
            tunnel: w167 -> [_ w191]
            frame #0 {
              w189 = string[] ["main", "Imaging Control Layer", "ProbeModel", "DProbe"]  # ws, mod, freq menu commands
              n63 = Format Into String(format string="IsTxChannelModulationEn %d" ("Format String"), w181) -> (resulting string=w188:string)  [unwired: 2 in, 1 out]
              n64 = Build Array (concatenate)(w189, w188) -> (w185:string[])
              n65 = Array Size(array=w185) -> (size(s)=w186:i32)
              n66 = Initialize Array(sgl 0.0 ("Element Data"), w186) -> (w184:sgl[])
              n67 = call "tcpCmdArrayToZ_modify.vi"("Delay (sec)"=w184, "error in (no error)"=w180, "Timeout (ms)"=w182, "Command array"=w185, "connection ID in"=w183) -> ("error out"=w179:errorcluster)  [unwired: 2 in, 4 out]
            }
            frame #1 {
              w209 = string[] ["main", "Hardware Control Layer", "Xp", "DImage"]  # ws, mod, freq menu commands
              n68 = case shown="0" w193 {
                selector: w193 -> [w210 w213 w222]
                tunnel: w204 -> [w212 w219 w226]
                tunnel: [w212 w218 w223] -> w203
                tunnel: [w211 w217 w224] -> w202
                tunnel: w201 -> [w211 w216 w225]
                tunnel: w200 -> [_ w215 _]
                tunnel: w199 -> [_ w214 w221]
                tunnel: [w210 w213 w222] -> w197
                tunnel: w192 -> [_ _ w227]
                tunnel: w191 -> [_ _ w220]
                frame Default {
                }
                frame 3 {
                  n69 = call "WF3.vi"("TxWaveformStyle"=w213, "TxFreqIndex"=w214, "BeamStyleIndex"=w215, "Timeout (ms)"=w216, "connection ID in"=w219) -> ("Timeout (ms) out"=w217:i32, "connection ID out"=w218:refnum<k5>)  [unwired: 5 in]
                }
                frame 0 {
                  n70 = case shown="\"Common\", 기본" w220 {
                    tunnel: w227 -> [w234 w241]
                    tunnel: w226 -> [w233 w240]
                    tunnel: w225 -> [w232 w239]
                    tunnel: [w231 w238] -> w224
                    tunnel: [w230 w237] -> w223
                    tunnel: w221 -> [w228 w235]
                    frame "Common", Default {
                      n71 = call "WF0_RLE.vi"("connection ID in"=w233, "TxPulseRleA"=w234, "Mode control"=enum32{"D-mode", "B-mode"}."D-mode", "Timeout (ms)"=w232, "TxFrequencyIndex"=w228) -> ("connection ID out"=w230:refnum<k5>, "Timeout (ms) out"=w231:i32)  [unwired: 1 in]
                    }
                    frame "Griffin" {
                      n72 = call "WF0_RLE_griffin.vi"("connection ID in"=w240, "TxPulseRleA"=w241, "Mode control"=enum32{"D-mode", "B-mode"}."D-mode", "Timeout (ms)"=w239, "TxFrequencyIndex"=w235) -> ("connection ID out"=w237:refnum<k5>, "Timeout (ms) out"=w238:i32)  [unwired: 1 in]
                    }
                  }
                }
              }
              n73 = Format Into String(format string="TxWaveformStyleA poke 0 %d" ("Format String"), w197) -> (resulting string=w196:string)  [unwired: 2 in, 1 out]
              n74 = Build Array (concatenate)(w209, w196) -> (w206:string[])
              n75 = Array Size(array=w206) -> (size(s)=w207:i32)
              n76 = Initialize Array(0.2 ("Element Data"), w207) -> (w205:dbl[])
              n77 = call "tcpCmdArrayToZ_modify.vi"("Delay (sec)"=w205, "error in (no error)"=w195, "Timeout (ms)"=w202, "Command array"=w206, "connection ID in"=w203) -> ("error out"=w194:errorcluster)  [unwired: 2 in, 4 out]
            }
          }
        }
      }
    }
    frame #6 {
      n78 = case shown="거짓" w242 {
        tunnel: w247 -> [w267 w276]
        tunnel: w246 -> [w266 _]
        tunnel: w245 -> [w265 w278]
        tunnel: w244 -> [w264 w277]
        tunnel: [w263 _] -> w243
        frame False {
          w251 = 100.0
          w260 = string[] ["main", "Imaging Control Layer", "ImageModel", "DImage"]  # TxElement, Cycle, PRF change
          n79 = Unbundle By Name(w267) -> ("numTxCycles"=w248:dbl, "numTxElements"=w261:i16)
          n80 = Multiply(x=w251, y=w248) -> (x*y=w252:dbl)
          n81 = Round To Nearest(number=w252) -> (nearest integer value=w250:dbl)
          n82 = Divide(x=w250, y=w251) -> (x/y=w249:dbl)
          n83 = Format Into String(format string="NumTxElementsA poke 0 %d" ("Format String"), w261) -> (resulting string=w253:string)  [unwired: 2 in, 1 out]
          n84 = Format Into String(format string="NumTxCyclesA poke 0 %f" ("Format String"), w249) -> (resulting string=w254:string)  [unwired: 2 in, 1 out]
          n85 = Build Array (concatenate)(w260, w253, w254) -> (w257:string[])
          n86 = Array Size(array=w257) -> (size(s)=w259:i32)
          n87 = Initialize Array(0.5 ("element"), w259) -> (w256:dbl[])
          n88 = call "tcpCmdArrayToZ_modify.vi"("Delay (sec)"=w256, "error in (no error)"=w266, "Timeout (ms)"=w264, "Command array"=w257, "connection ID in"=w265) -> ("error out"=w263:errorcluster)  [unwired: 2 in, 4 out]
        }
        frame True {
          w271 = string[] ["main", "Imaging Control Layer", "ImageModel", "DImage"]  # NumTxElements Change
          n89 = Unbundle By Name(w276) -> ("numTxElements"=w268:i16)
          n90 = Format Into String(format string="NumTxElementsA poke 0 %d" ("Format String"), w268) -> (resulting string=w270:string)  [unwired: 2 in, 1 out]
          n91 = Build Array (concatenate)(w271, w270) -> (w269:string[])
          n92 = Array Size(array=w269) -> (size(s)=w272:i32)
          n93 = Initialize Array(sgl 0.0 ("element"), w272) -> (w274:sgl[])
          n94 = call "tcpCmdArrayToZ_modify.vi"("Delay (sec)"=w274, "Timeout (ms)"=w277, "Command array"=w269, "connection ID in"=w278) -> ()  [unwired: 3 in, 5 out]
        }
      }
    }
    frame #7 {
      w287 = string[] ["main", "Imaging Control Layer", "ImageModel", "DImage"]  # PRF Feedback
      w291 = 100.0
      n95 = Unbundle By Name(w293) -> ("pulseRepetRate"=w289:dbl)
      n96 = Multiply(x=w291, y=w289) -> (x*y=w292:dbl)
      n97 = Round To Nearest(number=w292) -> (nearest integer value=w290:dbl)
      n98 = Divide(x=w290, y=w291) -> (x/y=w280:dbl)
      n99 = Format Into String(format string="SampleRateHz %f" ("Format String"), w280) -> (resulting string=w282:string)  [unwired: 2 in, 1 out]
      n100 = Build Array (concatenate)(w287, w282) -> (w288:string[])
      n101 = Array Size(array=w288) -> (size(s)=w286:i32)
      n102 = Initialize Array(0.4 ("element"), w286) -> (w284:dbl[])
      n103 = call "tcpCmdArrayToZ_modify.vi"("Delay (sec)"=w284, "Timeout (ms)"=w279, "Command array"=w288, "connection ID in"=w281) -> ()  [unwired: 3 in, 5 out]
    }
    frame #8 {
      n104 = case shown="\"Common\", 기본" w294 {
        tunnel: [w305 w306] -> w300
        frame "Common", Default {
          w305 = string[] ["main", "Hardware Control Layer", "Beamforming", "DImage"]  # Voltage menu commands
        }
        frame "K2" {
          w306 = string[] ["main", "Hardware Control Layer", "Fe", "DImage"]  # Voltage menu commands
        }
      }
      n105 = Format Into String(format string="TxFrequencyIndexA poke 0 %d" ("초기 문자열"), w297) -> (resulting string=w299:string)  [unwired: 2 in, 1 out]
      n106 = Build Array (concatenate)(w300, w299) -> (w298:string[])
      n107 = Array Size(array=w298) -> (size(s)=w304:i32)
      n108 = Initialize Array(0.4 ("element"), w304) -> (w302:dbl[])
      n109 = call "tcpCmdArrayToZ_modify.vi"("Delay (sec)"=w302, "Timeout (ms)"=w295, "Command array"=w298, "connection ID in"=w296) -> ()  [unwired: 3 in, 5 out]
    }
    frame #9 {
      n110 = Unbundle By Name(w308) -> ("IsCPAEn"=w312:i16)
      n111 = global read "Thermal_type.vi" "System \nSelection"() -> (w307:enum32{"Common", "Frosk", "Griffin", "K2"})
      n112 = case shown="\"Griffin\"" w307 {
        tunnel: w311 -> [w323 w334 _]
        tunnel: w310 -> [w322 w333 _]
        tunnel: w312 -> [w315 w326 _]
        tunnel: w309 -> [w313 w324 _]
        frame "K2" {
          w314 = string[] ["main", "Hardware Control Layer", "Fe", "DImage"]  # ws, mod, freq menu commands
          n113 = Format Into String(format string="IsCPAEn %d" ("Format String"), w315) -> (resulting string=w320:string)  [unwired: 2 in, 1 out]
          n114 = Build Array (concatenate)(w314, w320) -> (w317:string[])
          n115 = Array Size(array=w317) -> (size(s)=w319:i32)
          n116 = Initialize Array(0.4 ("element"), w319) -> (w316:dbl[])
          n117 = call "tcpCmdArrayToZ_modify.vi"("Delay (sec)"=w316, "error in (no error)"=w313, "Timeout (ms)"=w322, "Command array"=w317, "connection ID in"=w323) -> ()  [unwired: 2 in, 5 out]
        }
        frame "Griffin" {
          w325 = string[] ["main", "Hardware Control Layer", "Beamforming", "DImage"]  # ws, mod, freq menu commands
          n118 = Format Into String(format string="IsCPAEn %d" ("Format String"), w326) -> (resulting string=w331:string)  [unwired: 2 in, 1 out]
          n119 = Build Array (concatenate)(w325, w331) -> (w328:string[])
          n120 = Array Size(array=w328) -> (size(s)=w330:i32)
          n121 = Initialize Array(0.4 ("element"), w330) -> (w327:dbl[])
          n122 = call "tcpCmdArrayToZ_modify.vi"("Delay (sec)"=w327, "error in (no error)"=w324, "Timeout (ms)"=w333, "Command array"=w328, "connection ID in"=w334) -> ()  [unwired: 2 in, 5 out]
        }
        frame Default {
        }
      }
    }
    frame #10 {
      n123 = global read "Thermal_type.vi" "System \nSelection"() -> (w336:enum32{"Common", "Frosk", "Griffin", "K2"})
      n124 = case shown="\"K2\"" w336 {
        tunnel: w339 -> [_ w345 w358]
        tunnel: w338 -> [_ w344 w357]
        tunnel: w337 -> [_ w343 w356]
        tunnel: [0.0 w341 w354] -> w335
        frame "Common", Default {
        }
        frame "Griffin" {
          w342 = string[] ["main", "Hardware Control Layer", "Beamforming", "DImage", "IsCPAEn"]  # ws, mod, freq menu commands
          n125 = Array Size(array=w342) -> (size(s)=w350:i32)
          n126 = Initialize Array(0.0 ("원소"), w350) -> (w352:dbl[])
          n127 = call "tcpCmdArrayToZ_modify.vi"("Delay (sec)"=w352, "error in (no error)"=w344, "Timeout (ms)"=w343, "Command array"=w342, "connection ID in"=w345) -> ("Receive array"=w351:string[])  [unwired: 2 in, 4 out]
          n128 = Decrement(x=w350) -> (x-1=w348:i32)
          n129 = Index Array(array=w351, index=w348) -> (element=w349:string)
          n130 = Match Pattern(string=w349, regular expression="250 " ("정규식")) -> (after substring=w347:string)  [unwired: 1 in, 3 out]
          n131 = Fract/Exp String To Number(string=w347) -> (number=w341:dbl)  [unwired: 3 in, 1 out]
        }
        frame "K2" {
          w355 = string[] ["main", "Hardware Control Layer", "Fe", "DImage", "IsCPAEn"]  # ws, mod, freq menu commands
          n132 = Array Size(array=w355) -> (size(s)=w363:i32)
          n133 = Initialize Array(0.0 ("원소"), w363) -> (w365:dbl[])
          n134 = call "tcpCmdArrayToZ_modify.vi"("Delay (sec)"=w365, "error in (no error)"=w357, "Timeout (ms)"=w356, "Command array"=w355, "connection ID in"=w358) -> ("Receive array"=w364:string[])  [unwired: 2 in, 4 out]
          n135 = Decrement(x=w363) -> (x-1=w361:i32)
          n136 = Index Array(array=w364, index=w361) -> (element=w362:string)
          n137 = Match Pattern(string=w362, regular expression="250 " ("정규식")) -> (after substring=w360:string)  [unwired: 1 in, 3 out]
          n138 = Fract/Exp String To Number(string=w360) -> (number=w354:dbl)  [unwired: 3 in, 1 out]
        }
      }
    }
    frame #11 {
      w374 = 100.0
      # "SampleRateHz"
      # "PulseVoltage"
      # "TxFrequencyIndex"
      n139 = Unbundle By Name(w393) -> ("VTxIndex"=w392:i8, "elevAperIndex"=w391:i8, "txpgWaveformStyle"=w370:i8, "TxPulseRleA"=w378:string, "IsCPAEn"=w368:i16)
      n140 = call "Command_verification.vi"("connection ID"=w396, "System \nSelection"=w390, "Mode"="DProbe", "VTxIndex_In"=w392, "probeNumElevAper"=w385, "time out"=w395, "elevAperIndex"=w391, "TxpgWaveformStyle"=w370) -> ("Get_mea_condition"=w389:T4, "ElevAperSwitchDepth"=w383:sgl, "Result_RLE"=w369:bool, "RLE data"=w377:string, "Control_elevAperSwitch"=w388:bool)  [unwired: 3 in]
      n141 = Unbundle By Name(w394) -> ("isTxAperModulationEn"=w405:i16, "txpgWaveformStyle"=w404:i16, "numTxCycles"=w372:dbl, "numTxElements"=w403:i16)
      n142 = case shown="1, 기본" w385 {
        tunnel: w383 -> [w419 _]
        tunnel: w384 -> [w420 _]
        tunnel: [w420 w421] -> w381
        tunnel: [w419 w421] -> w382
        frame 2 {
        }
        frame 1, Default {
          w421 = sgl 0.0 ("Default Value 2")
        }
      }
      n143 = Unbundle By Name(w389) -> ("isTxAperModulationEn"=w402:i16, "txpgWaveformStyle"=w401:i16, "numTxCycles"=w400:dbl, "numTxElements"=w379:i16, "pulseRepetRate"=w399:dbl, "txFrequencyIndex"=w398:i32)
      n144 = Multiply(x=w374, y=w372) -> (x*y=w375:dbl)
      n145 = Round To Nearest(number=w375) -> (nearest integer value=w373:dbl)
      n146 = Divide(x=w373, y=w374) -> (x/y=w371:dbl)
      n147 = case shown="기본" w370 {
        tunnel: w378 -> [_ w418]
        tunnel: w377 -> [_ w417]
        tunnel: [TRUE w416] -> w376
        frame Default {
        }
        frame 0 {
          n148 = Equal?(x=w418, y=w417) -> (x = y?=w416:bool)
        }
      }
      n149 = case shown="거짓" w397 {
        tunnel: w413 -> [w439 _]
        tunnel: w412 -> [w438 w447]
        tunnel: [w437 w442] -> w407
        tunnel: [w436 w441] -> w406
        tunnel: w405 -> [w435 w449]
        tunnel: w404 -> [w424 w448]
        tunnel: w371 -> [w434 _]
        tunnel: w403 -> [w433 w446]
        tunnel: w402 -> [w432 w445]
        tunnel: w401 -> [w431 w444]
        tunnel: w400 -> [w430 _]
        tunnel: w379 -> [w429 w440]
        tunnel: w399 -> [w428 _]
        tunnel: w398 -> [w427 w443]
        tunnel: w382 -> [w426 _]
        tunnel: w381 -> [w425 _]
        tunnel: w368 -> [w423 _]
        tunnel: w367 -> [w422 _]
        frame False {
          n150 = Build Array(w435, w424, w434, w433, w439, w438, w425, w423) -> (w437:dbl[])
          n151 = Build Array(w432, w431, w430, w429, w428, w427, w426, w422) -> (w436:dbl[])
        }
        frame True {
          n152 = Build Array(w449, w448, w447, w446) -> (w442:i16[])
          n153 = Build Array(w445, w444, w443, w440) -> (w441:i32[])
        }
      }
      n154 = Equal?(x=w407, y=w406) -> (x = y?=w410:bool[])
      "All_param_veri" <- w410
      n155 = Array Size(array=w410) -> (size(s)=w411:i32)
      n156 = Boolean To (0,1)(Boolean=w410) -> (0, 1=w408:i16[])
      n157 = Add Array Elements(numeric array=w408) -> (sum=w409:i16)
      "Pass_count" <- w409
      n158 = Equal?(x=w409, y=w411) -> (x = y?=w387:bool)
      "veri_P/F" <- w387
      n159 = Compound Arithmetic op=AND(w387, w388, w376, w369) -> (w386:bool)
      "meas_temparature_Output" <- w394
      "error out" <- w414
    }
    frame #12 {
      w463 = 100.0
      # "Set voltage and volt supply channel"
      n160 = Unbundle By Name(w465) -> ("pulseVoltage"=w461:dbl)
      n161 = Unbundle By Name(w460) -> ("VTxIndex"=w459:i8, "SysPulserSelA"=w450:i16)
      n162 = Multiply(x=w463, y=w461) -> (x*y=w464:dbl)
      n163 = Round To Nearest(number=w464) -> (nearest integer value=w462:dbl)
      n164 = Divide(x=w462, y=w463) -> (x/y=w455:dbl)
      n165 = case shown="참" w451 {
        tunnel: w455 -> [w466 w468]
        tunnel: [w466 w467] -> w454
        frame False {
          # "PW"
        }
        frame True {
          # "CW"
          n166 = In Range and Coerce(upper limit=sgl 10.0, x=w468, lower limit=sgl 0.1) -> (coerced(x)=w467:dbl)  [unwired: 1 out]
        }
      }
      n167 = case shown="\"K2\"" w452 {
        tunnel: w459 -> [_ w486 w497]
        tunnel: w458 -> [w475 w492 w502]
        tunnel: w457 -> [w474 w487 w498]
        tunnel: w456 -> [w473 w491 w501]
        tunnel: w454 -> [w472 w485 w496]
        tunnel: [TRUE ("x = y?") w484 w494] -> w453
        tunnel: w451 -> [_ _ w500]
        tunnel: w450 -> [_ _ w493]
        frame "Common", "Frosk", Default {
          w482 = string[] ["main", "Hardware Control Layer", "Beamforming", "Common"]  # Voltage menu commands
          n168 = Format Into String(format string="PulseVoltageA poke %d %.2f" ("Format String"), i8 0 ("입력 1"), w472) -> (resulting string=w481:string)  [unwired: 2 in, 1 out]
          n169 = Build Array (concatenate)(w482, w481) -> (w477:string[])
          n170 = Array Size(array=w477) -> (size(s)=w480:i32)
          n171 = Initialize Array(0.4 ("element"), w480) -> (w478:dbl[])
          n172 = call "tcpCmdArrayToZ_modify.vi"("Delay (sec)"=w478, "error in (no error)"=w473, "Timeout (ms)"=w474, "Command array"=w477, "connection ID in"=w475) -> ()  [unwired: 2 in, 5 out]
        }
        frame "Griffin" {
          n173 = call "VTx_control_Juniper.vi"("VTx_Voltage"=w485, "VTxIndex_In"=w486, "error in (no error)"=w491, "VTx1_voltage"=93.0, "Timeout (ms)"=w487, "connection ID in"=w492) -> ("error out"=w488:errorcluster, "connection ID out"=w489:refnum<k5>)  [unwired: 4 in]
          n174 = call "Control_verify_voltage.vi"("Timeout (ms)"=w487, "에러 입력(에러 없음)"=w488, "VTx_Voltage"=w485, "VTxIndex_In"=w486, "TCP 네트워크 연결 입력"=w489) -> ("Verify_voltage"=w484:bool)  [unwired: 2 in, 4 out]
        }
        frame "K2" {
          n175 = call "VTx_control_K2.vi"("VTx_Voltage"=w496, "VTxIndex_In"=w497, "SystemPulerSelA"=w493, "error in (no error)"=w501, "CW/SCW"=w500, "Timeout (ms)"=w498, "connection ID in"=w502) -> ("error out"=w495:errorcluster, "connection ID out"=w499:refnum<k5>)  [unwired: 3 in]
          n176 = call "Control_verify_voltage.vi"("Timeout (ms)"=w498, "에러 입력(에러 없음)"=w495, "VTx_Voltage"=w496, "VTxIndex_In"=w497, "TCP 네트워크 연결 입력"=w499) -> ("Verify_voltage"=w494:bool)  [unwired: 2 in, 4 out]
        }
      }
    }
    frame #13 {
      n177 = And(x=w507, y=w506) -> (x .and. y?=w505:bool)
      n178 = case shown="참" w505 {
        tunnel: w509 -> [w513 _]
        tunnel: w508 -> [w512 _]
        tunnel: w504 -> [w511 w514]
        tunnel: [w510 w514] -> w503
        frame False {
          n179 = call "Control_Verify_Error.vi"("에러 입력(에러 없음)"=w511, "timeout (ms)"=w512, "TCP 네트워크 연결 입력"=w513) -> ("에러 출력"=w510:errorcluster)  [unwired: 2 in]
        }
        frame True {
        }
      }
      "error out 2" <- w503
    }
    frame #14 {
      n180 = global read "Thermal_type.vi" "Measurement Type"() -> (w515:enum32{"Volt", "SA"})
      n181 = call "Monitoring PRF.vi"("Measurement Type"=w515, "timeout (ms)"=w517, "TCP from Orchid in"=w518) -> ("PRF"=→"Actual PRF":dbl)  [unwired: 6 in, 1 out]
    }
    frame #15 {
      # "Doppler gate position disable"
      n182 = Format Into String(format string="value %d" ("Format String"), 0 ("입력 1")) -> (resulting string=w521:string)  [unwired: 2 in, 1 out]
      n183 = Build Array (concatenate)(string[] ["main", "debug", "Ic", "Ic Events", "Common Events", "PriorityModeChangeEvent opt"] ("ROI Minimum"), w521, string[] ["back", "Common Events", "PriorityModeChangeEvent"] ("ROI Minimum")) -> (w519:string[])
      n184 = Array Size(array=w519) -> ()  [unwired: 1 out]
      n185 = Initialize Array(sgl 0.0 ("element")) -> (w527:sgl[])  [unwired: 1 in]
      n186 = call "tcpCmdArrayToZ_modify.vi"("Delay (sec)"=w527, "Timeout (ms)"=w524, "Command array"=w519, "connection ID in"=w525) -> ()  [unwired: 3 in, 5 out]
    }
  }
